vi "Query Multi Eval Meas List SEM OBW Limit Check Results.vi"(8 "error in (no error)":errorcluster, 9 "Result Type (Current)":i32(ring) items=["Current", "Average", "Extreme"], 10 "Instance (1)":T1=1, 11 "VISA resource name":refnum<visa-resource-name>) -> (0 "error out":errorcluster, 1 "SEM OBW Limit Check Results":i32[](array[numeric]), 2 "Reliability":i32, 3 "VISA resource name out":refnum<visa-resource-name>)   [LabVIEW 2015, in "Rohde&Schwarz CMXP NR FR2 Measurement.lvlib"]
doc: "Returns the limit check results for the occupied bandwidth for all measured list mode segments.\n\nAttributes:\nRSCMXPNRFR2M_ATTR_QUERY_MULTI_EVAL_MEASUREMENT_LIST_SEM_OBW_AVERAGE_LIMIT_CHECK_RESULTS\nRSCMXPNRFR2M_ATTR_QUERY_MULTI_EVAL_MEASUREMENT_LIST_SEM_OBW_CURRENT_LIMIT_CHECK_RESULTS\nRSCMXPNRFR2M_ATTR_QUERY_MULTI_EVAL_MEASUREMENT_LIST_SEM_OBW_EXTREME_LIMIT_CHECK_RESULTS\n\nRemote-control commands:\nCALCulate:NRMMw:MEAS<i>:MEValuation:LIST:SEMask:OBW:AVERage?\nCALCulate:NRMMw:MEAS<i>:MEValuation:LIST:SEMask:OBW:CURRent?\nCALCulate:NRMMw:MEAS<i>:MEValuation:LIST:SEMask:OBW:EXTReme?"
uses:
  <instrlib>/Rohde&Schwarz CMXP NR FR2 Measurement/Rohde&Schwarz CMXP NR FR2 Measurement.lvlib
  <instrlib>/Rohde&Schwarz CMXP NR FR2 Measurement/Private/_Instance.ctl
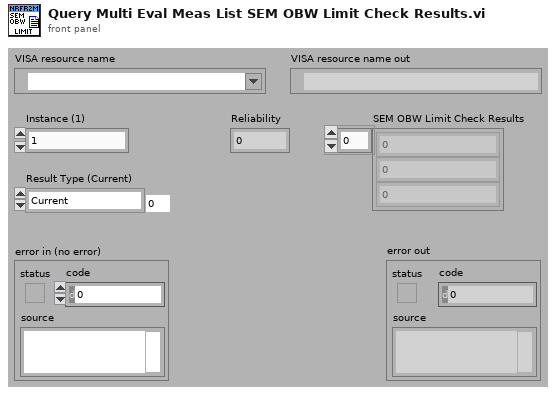
[diagram p1: front panel]
types:
  T1 = typedef "Rohde&Schwarz CMXP NR FR2 Measurement.lvlib/_Instance.ctl" = i32
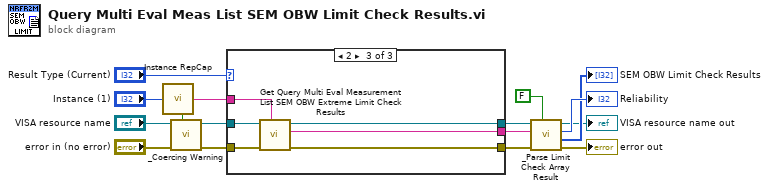
[diagram p0: block diagram]
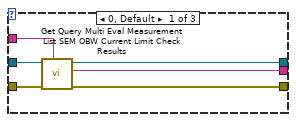
[diagram p2: hidden frame]
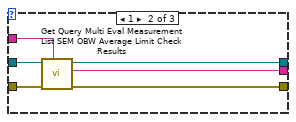
[diagram p3: hidden frame]
diagram:
  n1 = call <instrlib>:"Instance RepCap.vi"("Instance In"="Instance (1)") -> ("In Range?"=w14:bool, "RepCap Identifier Out"=w11:string)  [unwired: 1 in]
  n2 = call <instrlib>:"_Coercing Warning.vi"("In Range?"=w14, "error in (no error)"="error in (no error)", "VISA resource name"="VISA resource name") -> ("error out"=w12:errorcluster, "VISA resource name out"=w13:refnum<visa-resource-name>)  [unwired: 7 in]
  n3 = case shown="2" "Result Type (Current)" {
    tunnel: w13 -> [w22 w28 w34]
    tunnel: w12 -> [w21 w27 w33]
    tunnel: w11 -> [w20 w26 w32]
    tunnel: [w19 w25 w31] -> w9
    tunnel: [w18 w24 w30] -> w8
    tunnel: [w17 w23 w29] -> w7
    frame 0, Default {
      n4 = call "Get Query Multi Eval Measurement List SEM OBW Current Limit Check Results"("Repeated Capabilities"=w20, "error in (no error)"=w21, "instrument handle"=w22) -> ("error out"=w19:errorcluster, "Query Multi Eval Measurement List SEM OBW Current Limit Check Results"=w18:string, "instrument handle out"=w17:refnum<visa-resource-name>)  [unwired: 6 in]
    }
    frame 1 {
      n5 = call "Get Query Multi Eval Measurement List SEM OBW Average Limit Check Results"("Repeated Capabilities"=w26, "error in (no error)"=w27, "instrument handle"=w28) -> ("error out"=w25:errorcluster, "Query Multi Eval Measurement List SEM OBW Average Limit Check Results"=w24:string, "instrument handle out"=w23:refnum<visa-resource-name>)  [unwired: 6 in]
    }
    frame 2 {
      n6 = call "Get Query Multi Eval Measurement List SEM OBW Extreme Limit Check Results"("Repeated Capabilities"=w32, "error in (no error)"=w33, "instrument handle"=w34) -> ("error out"=w31:errorcluster, "Query Multi Eval Measurement List SEM OBW Extreme Limit Check Results"=w30:string, "instrument handle out"=w29:refnum<visa-resource-name>)  [unwired: 6 in]
    }
  }
  n7 = call <instrlib>:"_Parse Limit Check Array Result.vi"("error in (no error)"=w9, "Input String"=w8, "VISA resource name"=w7, "Out of tolerance? (F)"=FALSE) -> ("error out"=→"error out":errorcluster, "Results"=→"SEM OBW Limit Check Results":i32[], "Reliability"=→"Reliability":i32, "VISA resource name out"=→"VISA resource name out":refnum<visa-resource-name>)  [unwired: 3 in]
